vi "Get_Array_Subset.vi"(5 "String Array In":string[](array[string]), 6 "Subset Name":string) -> (0 "index after match":i32, 1 "Array Subset Out":string[](array[string]), 2 "Empty Subset?":bool, 3 "Length before match":i32, 4 "First Element":string)   [LabVIEW 2020]
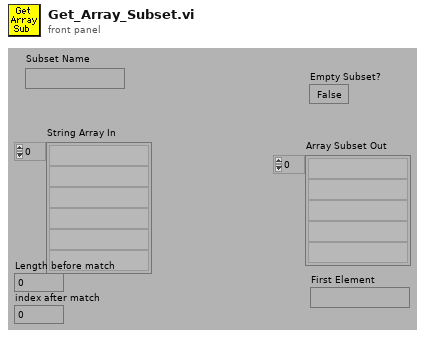
[diagram p1: front panel]
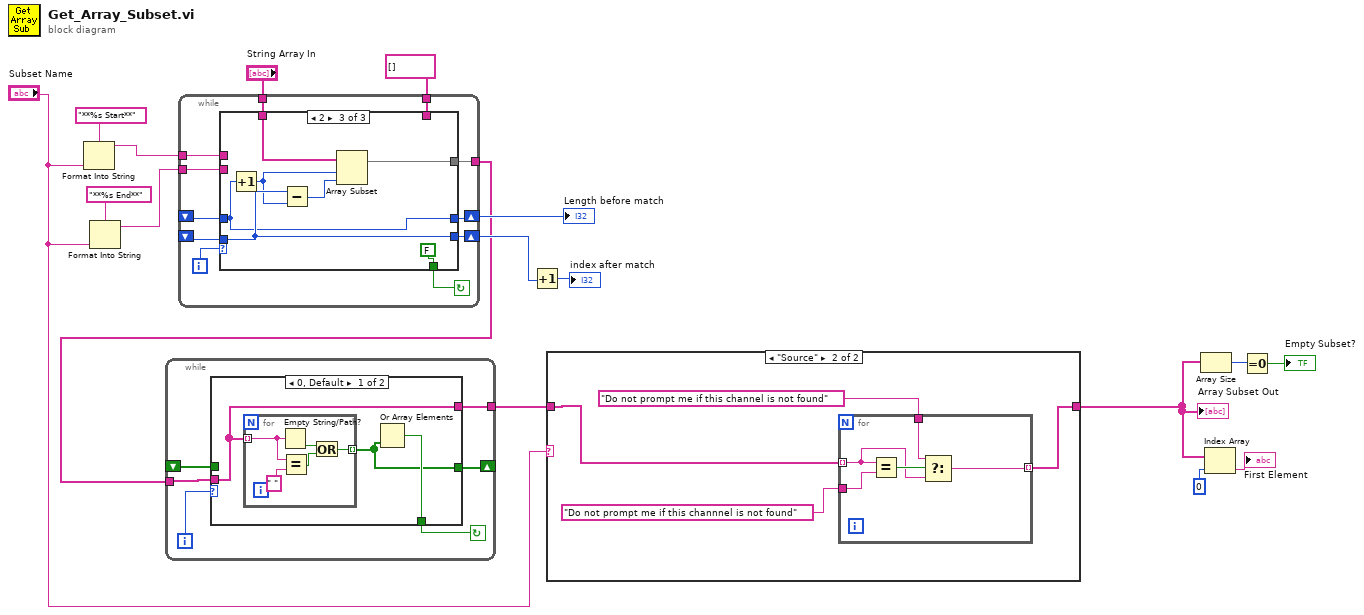
[diagram p0: block diagram]
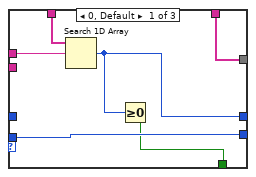
[diagram p3: hidden frame]
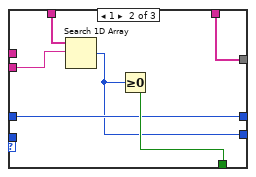
[diagram p4: hidden frame]
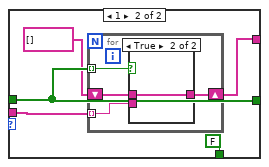
[diagram p5: hidden frame]
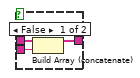
[diagram p6: hidden frame]
diagram:
  n1 = Format Into String(format string="**%s Start**" ("Format String"), "Subset Name") -> (resulting string=w14:string)  [unwired: 2 in, 1 out]
  n2 = Format Into String(format string="**%s End**" ("Format String"), "Subset Name") -> (resulting string=w12:string)  [unwired: 2 in, 1 out]
  n3 = while {
    tunnel: w12 -> [w19]
    shift-left: _ -> [w21]
    shift-right: [w20] -> w8
    shift-left: _ -> [w18]
    shift-right: [w22] -> w9
    tunnel: string[] [] ("Array Subset Out") -> [w23]
    tunnel: [w24] -> w6
    tunnel: w14 -> [w27]
    tunnel: "String Array In" -> [w28]
    i -> [w26]
    stop <- w25 continue-if-true
    n4 = case shown="2" w26 {
      tunnel: w28 -> [w34 w40 w43]
      tunnel: w27 -> [w33 _ _]
      tunnel: [w29 w38 FALSE] -> w25
      tunnel: [w32 w39 w44] -> w24
      tunnel: w23 -> [w32 w39 _]
      tunnel: [w30 w36 w42] -> w22
      tunnel: w21 -> [w31 _ w46]
      tunnel: [w31 w35 w46] -> w20
      tunnel: w19 -> [_ w37 _]
      tunnel: w18 -> [_ w36 w42]
      frame 0, Default {
        n5 = Search 1D Array(1D array=w34, element=w33) -> (index of element=w30:i32)  [unwired: 1 out]
        n6 = Greater Or Equal To 0?(x=w30) -> (x >= 0?=w29:bool)
      }
      frame 1 {
        n7 = Search 1D Array(1D array=w40, element=w37) -> (index of element=w35:i32)  [unwired: 1 out]
        n8 = Greater Or Equal To 0?(x=w35) -> (x >= 0?=w38:bool)
      }
      frame 2 {
        n9 = Increment(x=w42) -> (x+1=w41:i32)
        n10 = Subtract(x=w46, y=w41) -> (x-y=w47:i32)
        n11 = Array Subset(array=w43, index=w41, length=w47) -> (w44:string[])
      }
    }
  }
  "Length before match" <- w9
  n12 = while {
    shift-left: _ -> [w48]
    shift-right: [w49] -> _
    tunnel: [w50] -> w1
    tunnel: w6 -> [w52]
    i -> [w53]
    stop <- w51 continue-if-true
    n13 = case shown="0, Default" w53 {
      tunnel: w52 -> [w55 w63]
      tunnel: [w56 FALSE] -> w51
      tunnel: [w55 w66] -> w50
      tunnel: [w54 w65] -> w49
      tunnel: w48 -> [_ w65]
      frame 0, Default {
        n14 = for {
          tunnel: w55 -> [w60] mode=indexing
          tunnel: [w57] -> w54 mode=indexing
          n15 = Empty String/Path?(string/path=w60) -> (empty?=w58:bool)
          n16 = Equal?(x=w60, y=" ") -> (x = y?=w59:bool)
          n17 = Or(x=w58, y=w59) -> (x .or. y?=w57:bool)
        }
        n18 = Or Array Elements(Boolean array=w54) -> (logical OR=w56:bool)
      }
      frame 1 {
        n19 = for {
          shift-right: [w69] -> w66
          shift-left: string[] [] -> [w68]
          tunnel: w65 -> [w70] mode=indexing
          tunnel: w63 -> [w67] mode=indexing
          n20 = case shown="True" w70 {
            tunnel: [w72 w74] -> w69
            tunnel: w68 -> [w73 w74]
            tunnel: w67 -> [w71 _]
            frame False {
              n21 = Build Array (concatenate)(w73, w71) -> (w72:string[])
            }
            frame True {
            }
          }
        }
      }
    }
  }
  n22 = Increment(x=w8) -> (x+1=→"index after match":i32)
  n23 = case shown="\"Source\"" "Subset Name" {
    tunnel: [w75 w76] -> w2
    tunnel: w1 -> [w75 w79]
    frame Default {
    }
    frame "Source" {
      n24 = for {
        tunnel: w79 -> [w81] mode=indexing
        tunnel: "Do not prompt me if this channnel is not found" -> [w84]
        tunnel: "Do not prompt me if this channel is not found" -> [w82]
        tunnel: [w80] -> w76 mode=indexing
        n25 = Equal?(x=w81, y=w84) -> (x = y?=w83:bool)
        n26 = Select(t=w82, s=w83, f=w81) -> (s? t:f=w80:string)
      }
    }
  }
  "Array Subset Out" <- w2
  n27 = Array Size(array=w2) -> (size(s)=w11:i32)
  n28 = Index Array(array=w2, index=0 ("Index")) -> (element=→"First Element":string)
  n29 = Equal To 0?(x=w11) -> (x = 0?=→"Empty Subset?":bool)
